vi "InstrumentationU6Mk2.2.vi"() -> ()   [LabVIEW 2021]
panel:
  in  "stop":bool
  out "P-CombChamb":dbl(graph)
  out "P-Injector":dbl(graph)
  out "P-RunTank":dbl(graph)
  out "P-N2Flow":dbl(graph)
  out "P-N20Flow":dbl(graph)
  out "L-RunTank 2":dbl(graph)
  out "L-Thrust":dbl(graph)
  out "T-RunTank":dbl(graph)
  out "T-PoCombust":dbl(graph)
  out "T-Combustion":dbl(graph)
  out "T-Injector":dbl(graph)
  in  "Log Values":bool
  in  "file name":string
  in  "file path":path
  in  "Binary":bool
  in  "SettlingFactor":i32
  out "Values Read":dbl[](array[numeric]) format="%.6f"
  out "Error Message":string
  in  "Resolution":i32
  out "error out":errorcluster
  # "Aquires multiple analog input channels over USB from the first found U6.\n\nThis uses eAddGoGet from the UD driver, rather than the LabVIEW utility AddS-Go-Get.vi.  The utility\nVI has better/easier error handling and is normally preferred, but eAddGoGet is a single call to the UD driver\nso often preferred if you will have parallel driver calls to the same handle within the same thread (none of\nour examples do this)."
  # "LJ_rgBIP10V\nLJ_rgBIP1V\nLJ_rgBIPP1V\nLJ_rgBIPP01V"
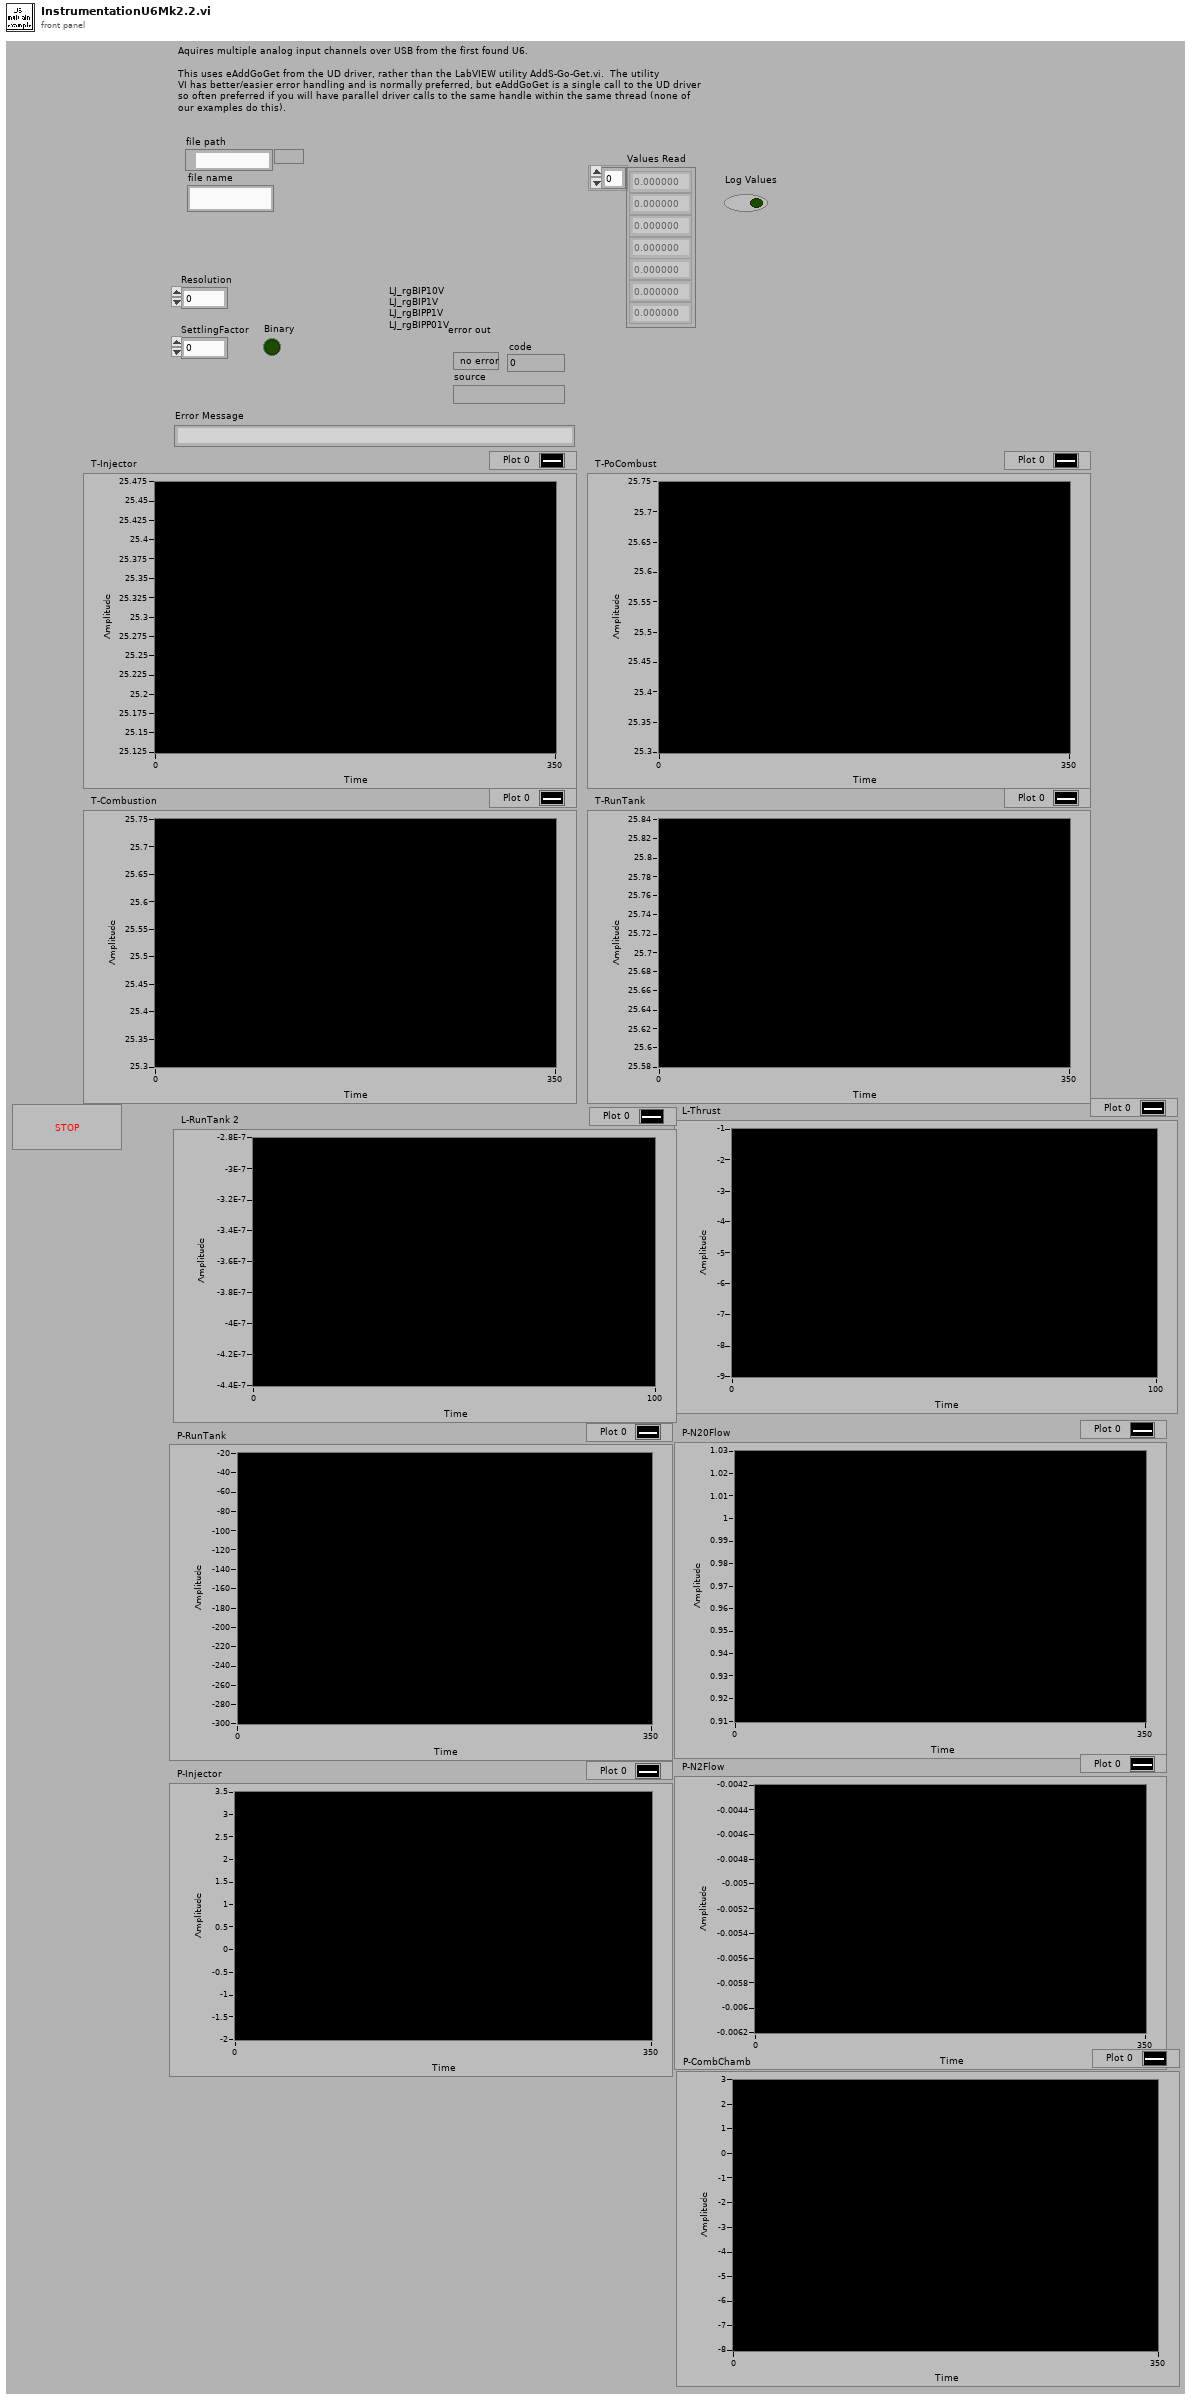
[diagram p1: front panel]
types:
  T1 = enum16{"open", "open or create", "create or replace", "create", "open (read-only)"}
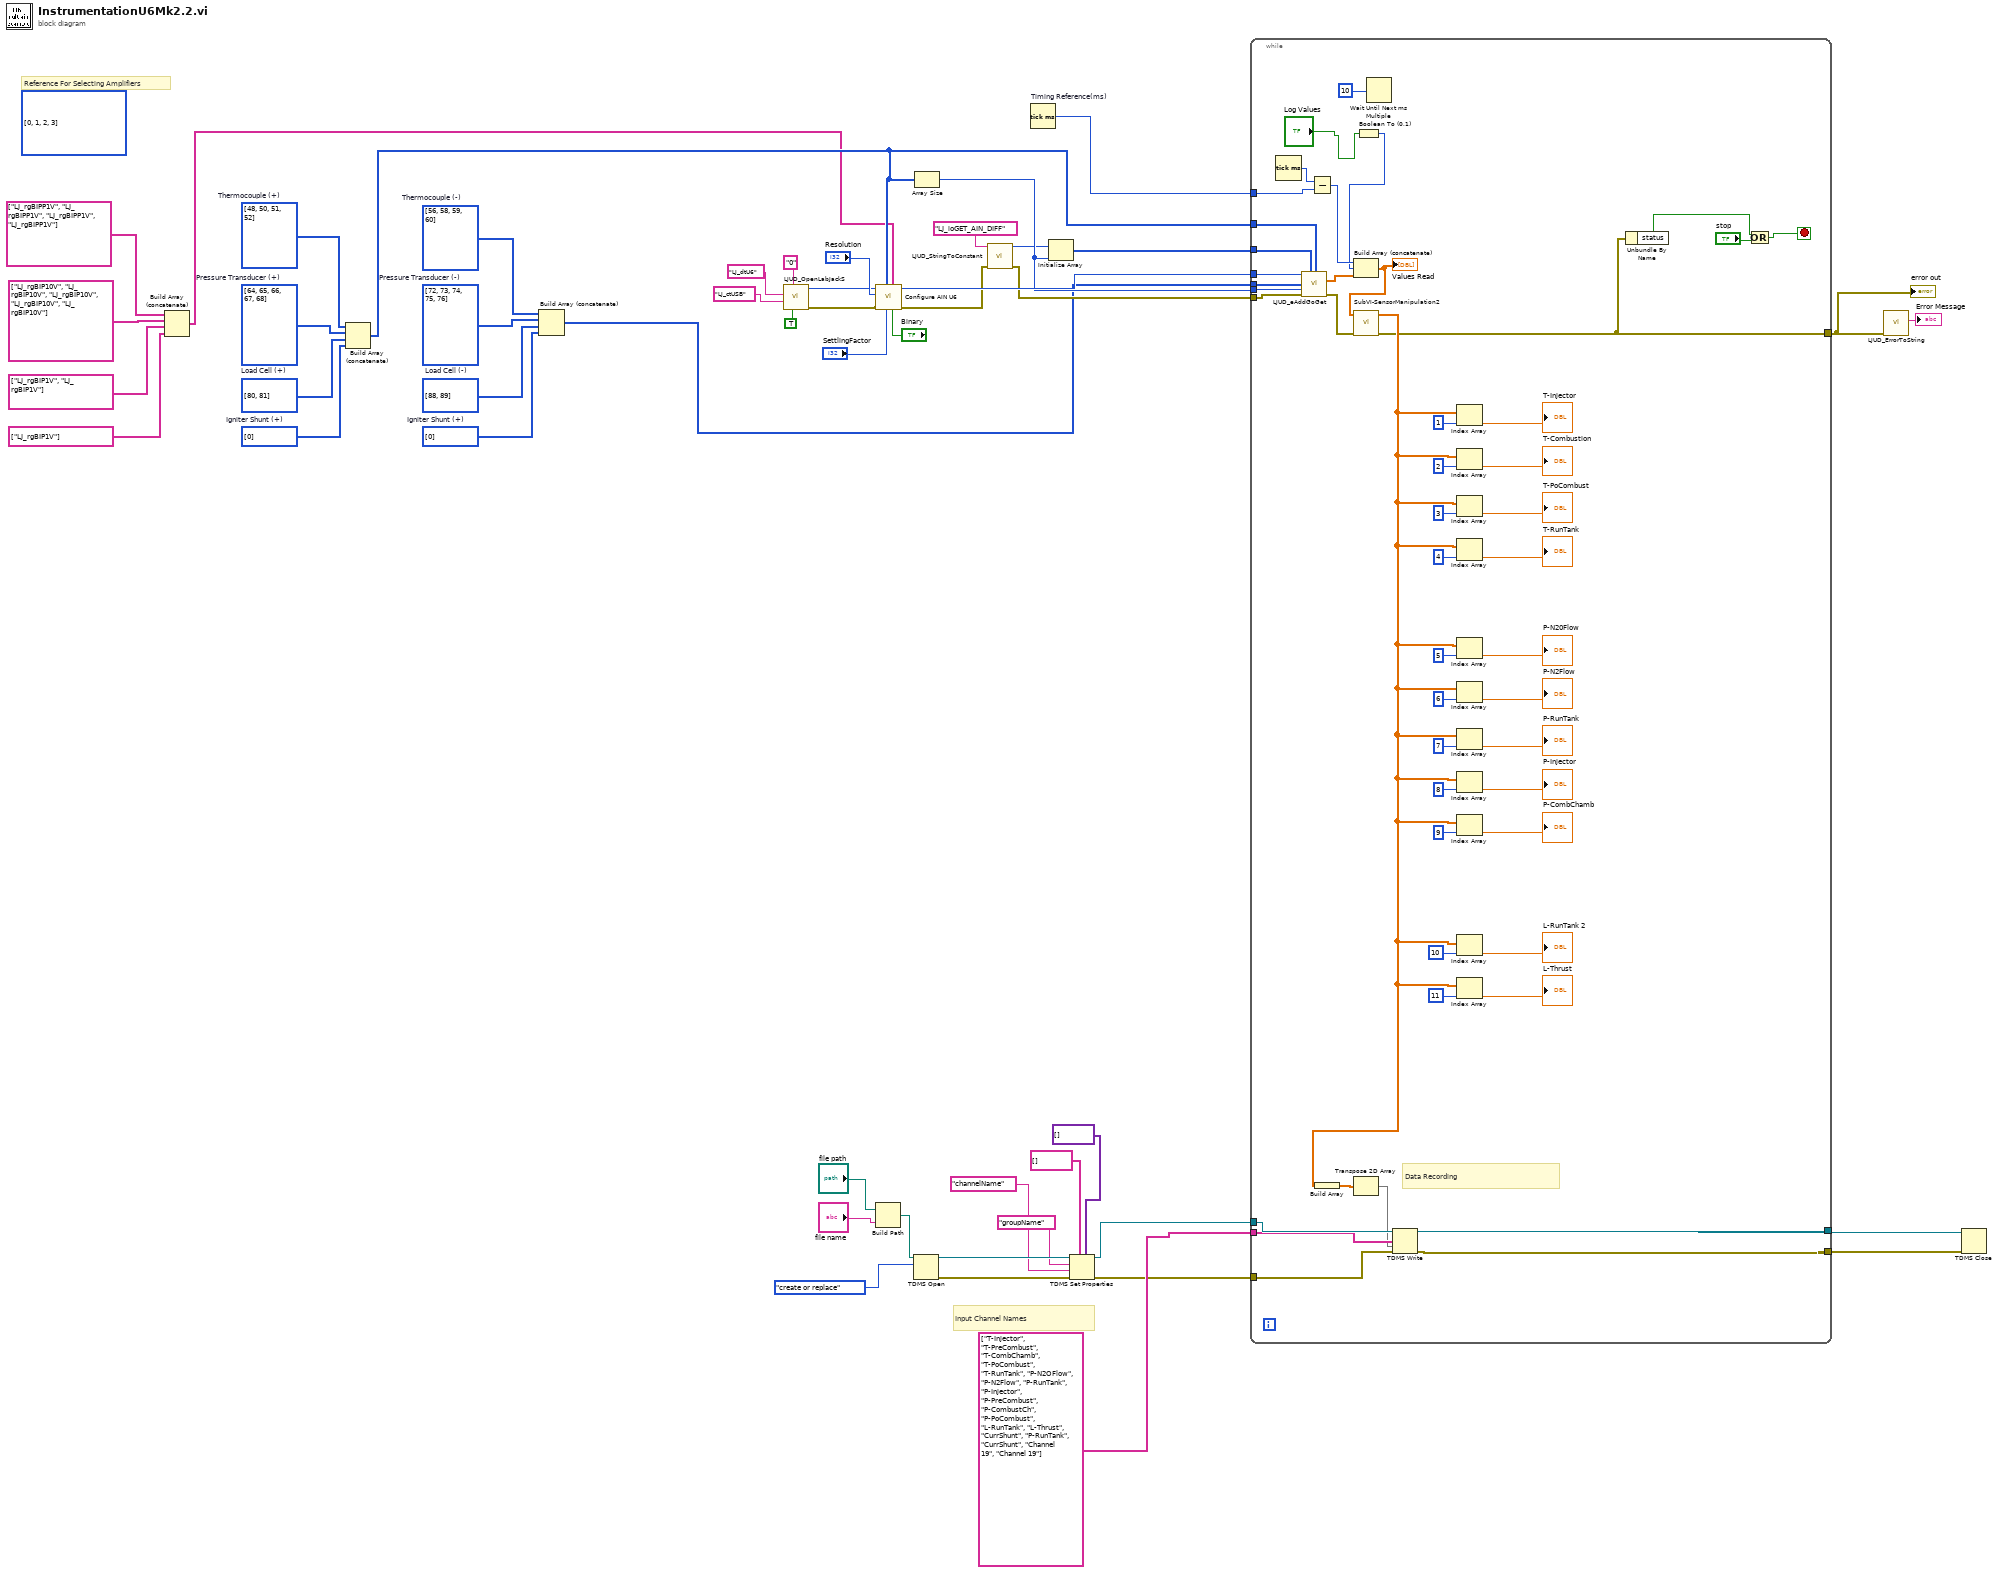
[diagram p0: block diagram]
diagram:
  w2 = i32[] [0]  # Igniter Shunt (+)
  w1 = i32[] [0]  # Igniter Shunt (+)
  w5 = i32[] [88, 89]  # Load Cell (-)
  w6 = i32[] [80, 81]  # Load Cell (+)
  (unwired) u8[] [0, 1, 2, 3] items=["LJ_rgBIP10V", "LJ_rgBIP1V", "LJ_rgBIPP1V", "LJ_rgBIPP01V"] ("Range Constants")
  w7 = i32[] [72, 73, 74, 75, 76]  # Pressure Transducer (-)
  w9 = i32[] [64, 65, 66, 67, 68]  # Pressure Transducer (+)
  w8 = i32[] [56, 58, 59, 60]  # Thermocouple (-)
  w10 = i32[] [48, 50, 51, 52]  # Thermocouple (+)
  # "Reference For Selecting Amplifiers"
  # "Input Channel Names"
  n1 = Build Array (concatenate)(string[] ["LJ_rgBIPP1V", "LJ_rgBIPP1V", "LJ_rgBIPP1V", "LJ_rgBIPP1V"] ("Ranges"), string[] ["LJ_rgBIP10V", "LJ_rgBIP10V", "LJ_rgBIP10V", "LJ_rgBIP10V", "LJ_rgBIP10V"] ("Ranges"), string[] ["LJ_rgBIP1V", "LJ_rgBIP1V"] ("Ranges"), string[] ["LJ_rgBIP1V"] ("Ranges")) -> (w15:string[])
  n2 = Build Array (concatenate)(w10, w9, w6, w1) -> (w17:i32[])
  n3 = Build Array (concatenate)(w8, w7, w5, w2) -> (w16:i32[])
  n4 = call "LJUD_OpenLabJackS.vi"("FirstFound"=TRUE, "Address"="0", "ConnectionType"="LJ_ctUSB", "DeviceType"="LJ_dtU6") -> ("error out"=w42:errorcluster, "Handle"=w43:i32)  [unwired: 5 in, 1 out]
  n5 = Build Path(base path="file path", name or relative path="file name") -> (appended path=w28:path)
  n6 = call "Configure AIN U6.vi"("Binary"="Binary", "Ranges"=w15, "SettlingFactor"="SettlingFactor", "Positive Channels"=w17, "error in"=w42, "Resolution"="Resolution", "Handle In"=w43) -> ("error out"=w39:errorcluster, "Handle Out"=w48:i32)  [unwired: 3 in]
  n7 = TDMS Open(10:T1."create or replace" ("operation (0:open)"), 11:w28) -> (0:w33:errorcluster, 3:w32:refnum<k34>)  [unwired: 5 in]
  n8 = Array Size(array=w17) -> (size(s)=w37:i32)
  n9 = call "LJUD_StringToConstant.vi"("error in"=w39, "String"="LJ_ioGET_AIN_DIFF" ("IOType")) -> ("error out"=w18:errorcluster, "Constant Number"=w36:i32)  [unwired: 8 in]
  n10 = Tick Count (ms) "Timing Reference(ms)"() -> (millisecond timer value=w34:u32)
  n11 = Initialize Array(w36, w37) -> (w35:i32[])
  n12 = TDMS Set Properties(5:variant[] [] ("property values"), 7:string[] [] ("property names"), 8:w33, 9:"channelName" ("channel name"), 10:"groupName" ("group name"), 11:w32) -> (0:w21:errorcluster, 3:w23:refnum<k34>)  [unwired: 2 out]
  n13 = while {
    tunnel: w48 -> [w98]
    tunnel: w16 -> [w97]
    tunnel: w37 -> [w96]
    tunnel: w35 -> [w95]
    tunnel: w34 -> [w93]
    tunnel: w17 -> [w69]
    tunnel: w23 -> [w91]
    tunnel: string[] ["T-Injector", "T-PreCombust", "T-CombChamb", "T-PoCombust", "T-RunTank", "P-N2OFlow", "P-N2Flow", "P-RunTank", "P-Injector", "P-PreCombust", "P-CombustCh", "P-PoCombust", "L-RunTank", "L-Thrust", "CurrShunt", "P-RunTank", "CurrShunt", "Channel 19", "Channel 19"] -> [w90]
    tunnel: w21 -> [w89]
    tunnel: [w88] -> w20
    tunnel: [w87] -> w19
    tunnel: w18 -> [w79]
    tunnel: [w50] -> w13
    stop <- w51 stop-if-true
    # "Data Recording"
    n14 = Tick Count (ms)() -> (millisecond timer value=w94:u32)
    n15 = call "LJUD_eAddGoGet.vi"("Handle In"=w98, "aIOTypes"=w95, "aChannels"=w69, "ax1s"=w97, "NumRequests"=w96, "error in"=w79) -> ("Values Read"=w83:dbl[], "error out"=w80:errorcluster)  [unwired: 4 in, 4 out]
    n16 = Subtract(x=w94, y=w93) -> (x-y=w92:u32)
    n17 = Boolean To (0,1)(Boolean="Log Values") -> (0, 1=w82:i16)
    n18 = Build Array (concatenate)(w92, w82, w83) -> (w81:dbl[])
    "Values Read" <- w81
    n19 = call "SubVI-SensorManipulation2.vi"("error in"=w80, "Array in"=w81) -> ("error out"=w50:errorcluster, "Array out"=w54:dbl[])  [unwired: 8 in]
    n20 = Build Array(w54) -> (w85:dbl[][])
    n21 = Transpose 2D Array(2D array=w85) -> (transposed array=w84:dbl[][])
    n22 = Wait Until Next ms Multiple(millisecond multiple=u32 10) -> ()  [unwired: 1 out]
    n23 = TDMS Write(0:w91, 7:w90, 9:w84, 11:w89) -> (4:w87:refnum<k34>, 15:w88:errorcluster)  [unwired: 2 in, 2 out]
    n24 = Index Array(array=w54, index=1) -> (element=→"T-Injector":dbl)
    n25 = Index Array(array=w54, index=2) -> (element=→"T-Combustion":dbl)
    n26 = Index Array(array=w54, index=3) -> (element=→"T-PoCombust":dbl)
    n27 = Index Array(array=w54, index=4) -> (element=→"T-RunTank":dbl)
    n28 = Index Array(array=w54, index=5) -> (element=→"P-N20Flow":dbl)
    n29 = Index Array(array=w54, index=6) -> (element=→"P-N2Flow":dbl)
    n30 = Index Array(array=w54, index=7) -> (element=→"P-RunTank":dbl)
    n31 = Index Array(array=w54, index=8) -> (element=→"P-Injector":dbl)
    n32 = Index Array(array=w54, index=9) -> (element=→"P-CombChamb":dbl)
    n33 = Index Array(array=w54, index=10) -> (element=→"L-RunTank 2":dbl)
    n34 = Index Array(array=w54, index=11) -> (element=→"L-Thrust":dbl)
    n35 = Unbundle By Name(w50) -> ("status"=w52:bool)
    n36 = Or(x=w52, y="stop") -> (x .or. y?=w51:bool)
  }
  "error out" <- w13
  n37 = call "LJUD_ErrorToString.vi"("error in"=w13) -> ("String"=→"Error Message":string)  [unwired: 10 in]
  n38 = TDMS Close(8:w20, 11:w19) -> ()  [unwired: 2 out]
